vi "Test App Prefix Update is Propagated to Owned Processes.vi"(8 "error in (no error)":errorcluster, 11 "Application Test in":refnum<class "Application Dev Test.lvclass">) -> (0 "error out":errorcluster, 3 "Application Test out":refnum<class "Application Dev Test.lvclass">)   [LabVIEW 2020, in "Application Dev Test.lvclass"]
uses:
  Application Dev Test.lvclass
  C:/Program Files (x86)/National Instruments/LabVIEW 2020/vi.lib/Astemes/LUnit/Test Case.lvclass
  source/Framework/Application/Application.lvclass
  C:/Git/astemes-triarc-framework/source/Framework/Process/Process.lvclass
  source/Framework/Process/Process.lvclass
  source/Framework/Process/Process.lvclass/Process.ctl
  source/Framework/Application/Application.lvclass/Application.ctl
  <vilib>/Astemes/LUnit/Test Case.lvclass/Test Case.ctl
  <vilib>/Astemes/LUnit/LUnit Assertion Result.lvclass/LUnit Assertion Result.ctl
  <vilib>/Astemes/LUnit/LUnit Test Case Result.lvclass/LUnit Test Case Result.ctl
  <vilib>/Astemes/LUnit/LUnit Method Result.lvclass/LUnit Method Result.ctl
  source/Framework/Application/Private/Add Process to Map.vi
  source/Framework/Application/Private/Start Idle Processes if Running.vi
  source/Framework/Application/Private/Throw Error If Process Already in App.vi
  source/Framework/Process/Protected/Messaging/Enqueue Message.vi
  source/Framework/Process/Public/Lifecycle/Get Lifecycle State.vi
  source/Framework/Process/Protected/SubVIs/Set Context.vi
  source/Framework/Application/Private/Retrieve Process from App.vi
  source/Framework/Application/Private/Parse Process Name.vi
  source/Framework/Application/Private/Get Process from Map.vi
  <vilib>/Astemes/LUnit/Palette/Pass If Equal.vi/cbf50e99-f124-4847-863a-8e9794d3dede.vi
  source/Framework/Process/Private/SubVIs/Wait for finish.vi
  source/Framework/Process/Private/SubVIs/Set Lifecycle State.vi
  source/Framework/Process/Private/SubVIs/Handle Debug Data.vi
  <vilib>/Utility/error.llb/Clear Errors.vi
  source/Framework/Process/Public/Lifecycle/Leave Process Loop.vi
  source/Framework/Process/Protected/Messaging/Request Message.vi
  <vilib>/AdvancedString/Delimited String to 1D String Array.vi
  <vilib>/Astemes/LUnit/Palette/Pass.vi
  <vilib>/Astemes/LUnit/Palette/Fail.vi
  <vilib>/Astemes/LUnit/Compare Variants.vi
  <vilib>/Astemes/LUnit/Describe Comparison.vi
  <vilib>/Astemes/LUnit/Set Assertion Type.vi
  source/Framework/Logging/Log Debug.vi
  <vilib>/AdvancedString/1D String Array to Delimited String.vi
  <vilib>/Utility/High Resolution Relative Seconds.vi
  source/Framework/Process/Private/SubVIs/Enqueue Request Message.vi
  <vilib>/Astemes/LUnit/Add test result.vi
  <vilib>/Astemes/LUnit/LUnit Write Passed.vi
  <vilib>/Astemes/LUnit/LUnit Write Message.vi
  <vilib>/Astemes/LUnit/LUnit Write Description.vi
  <vilib>/Astemes/LUnit/Variant to string.vi
  <vilib>/Astemes/LUnit/LUnit Write Assertion Type.vi
  <vilib>/Astemes/LUnit/LUnit Record Assertion Result.vi
  <vilib>/Astemes/LUnit/LUnit Aggregate Assertion Results.vi
  <vilib>/Astemes/LUnit/Assertion Result/LUnit Read Status.vi
  <vilib>/Astemes/LUnit/LUnit Read Message.vi
  <vilib>/Astemes/LUnit/LUnit Read Description.vi
  <vilib>/Astemes/LUnit/Method Result/LUnit Merge Status.vi
  <vilib>/Astemes/LUnit/LUnit Concatenate result strings.vi
  <vilib>/Utility/error.llb/Error Cluster From Error Code.vi
  source/Framework/Process/Private/SubVIs/Wait for Response Message.vi
  <vilib>/Utility/Data Type/Get Type Information.vi
  <vilib>/Utility/LVClass/Get LV Class Name.vi
  <vilib>/Astemes/LUnit/LUnit Assertion Result.lvclass
  Application Dev Test.lvclass/Application Dev Test.ctl
  <vilib>/Astemes/LUnit/Test Case.lvclass
  source/Framework Test Suite/Support/Framework Test Support.lvlib
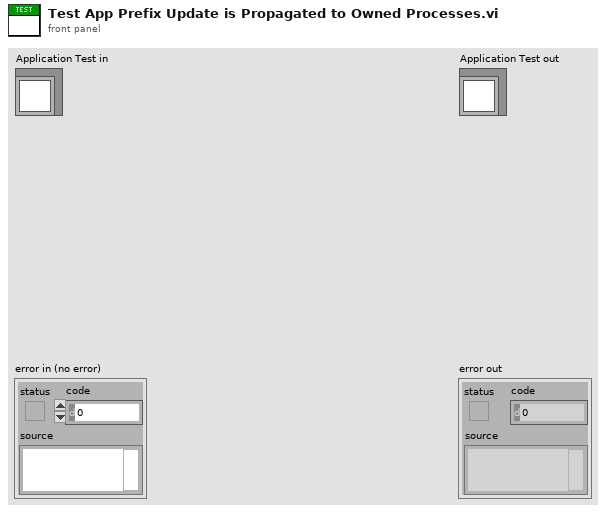
[diagram p1: front panel]
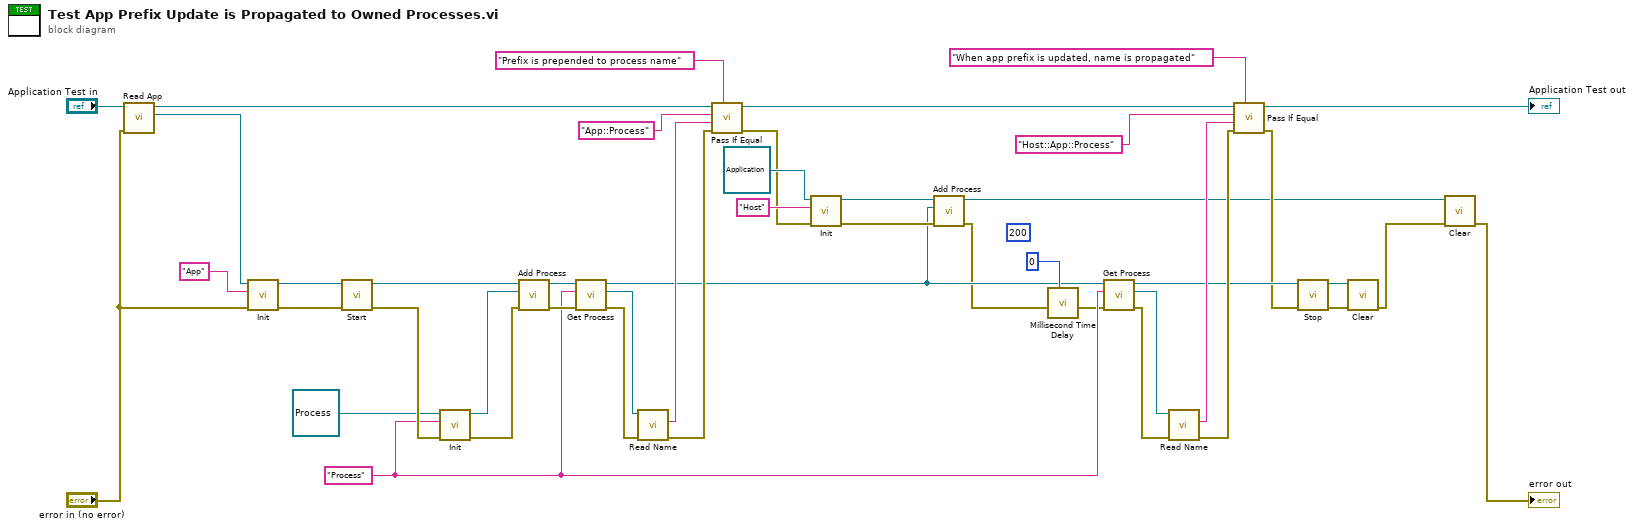
[diagram p0: block diagram]
diagram:
  (unwired) u32 200 ("milliseconds to wait")
  w21 = "Process" ("Name")
  n1 = call "Read App.vi"("error in (no error)"="error in (no error)", "Application Test In"="Application Test in") -> ("App out"=w12:refnum<class "Application.lvclass">, "Application Test Out"=w44:refnum<class "Application Dev Test.lvclass">)  [unwired: 7 in, 1 out]
  n2 = call-dynamic "Init.vi"("error in (no error)"="error in (no error)", "Name"="App", "Process In"=w12) -> ("error out"=w41:errorcluster, "Process Out"=w42:refnum<class "Application.lvclass">)  [unwired: 7 in]
  n3 = call "Start.vi"("error in (no error)"=w41, "Process In"=w42) -> ("error out"=w32:errorcluster, "Process Out"=w40:refnum<class "Application.lvclass">)  [unwired: 7 in, 1 out]
  n4 = call-dynamic "Init.vi"("error in (no error)"=w32, "Name"=w21, "Process In"=refnum<class "Process.lvclass"> refnum) -> ("error out"=w31:errorcluster, "Process Out"=w36:refnum<class "Process.lvclass">)  [unwired: 7 in]
  n5 = call "Add Process.vi"("error in (no error)"=w31, "Process"=w36, "Application In"=w40) -> ("error out"=w35:errorcluster, "Application Out"=w39:refnum<class "Application.lvclass">)  [unwired: 7 in]
  n6 = call "Get Process.vi"("error in (no error)"=w35, "Process Name"=w21, "Application In"=w39) -> ("error out"=w29:errorcluster, "App Process"=w30:refnum<class "Process.lvclass">, "Application Out"=w4:refnum<class "Application.lvclass">)  [unwired: 6 in]
  n7 = call "Read Name.vi"("error in (no error)"=w29, "Process In"=w30) -> ("error out"=w28:errorcluster, "Qualified Name"=w27:string)  [unwired: 6 in, 2 out]
  n8 = call <vilib>:"Pass If Equal.vi"("Description"="Prefix is prepended to process name", "error in (no error)"=w28, "Actual"=w27, "Expected"="App::Process", "LUnit Test Case In"=w44) -> ("error out"=w9:errorcluster, "LUnit Test Case Out"=w34:refnum<class "Application Dev Test.lvclass">)  [unwired: 5 in]
  n9 = call-dynamic "Init.vi"("error in (no error)"=w9, "Name"="Host" ("Prefix"), "Process In"=refnum<class "Application.lvclass"> refnum ("Rig In")) -> ("error out"=w7:errorcluster, "Process Out"=w8:refnum<class "Application.lvclass">)  [unwired: 7 in]
  n10 = call "Add Process.vi"("error in (no error)"=w7, "Process"=w4, "Application In"=w8) -> ("error out"=w3:errorcluster, "Application Out"=w6:refnum<class "Application.lvclass">)  [unwired: 7 in]
  n11 = call "Millisecond Time Delay.vi"("milliseconds to wait"=u32 0, "error in (no error)"=w3) -> ("error out"=w17:errorcluster)  [unwired: 7 in]
  n12 = call "Get Process.vi"("error in (no error)"=w17, "Process Name"=w21, "Application In"=w4) -> ("error out"=w23:errorcluster, "App Process"=w24:refnum<class "Process.lvclass">, "Application Out"=w14:refnum<class "Application.lvclass">)  [unwired: 6 in]
  n13 = call "Read Name.vi"("error in (no error)"=w23, "Process In"=w24) -> ("error out"=w18:errorcluster, "Qualified Name"=w22:string)  [unwired: 6 in, 2 out]
  n14 = call <vilib>:"Pass If Equal.vi"("Description"="When app prefix is updated, name is propagated", "error in (no error)"=w18, "Actual"=w22, "Expected"="Host::App::Process", "LUnit Test Case In"=w34) -> ("error out"=w13:errorcluster, "LUnit Test Case Out"=→"Application Test out":refnum<class "Application Dev Test.lvclass">)  [unwired: 5 in]
  n15 = call "Stop.vi"("error in (no error)"=w13, "Process In"=w14) -> ("error out"=w37:errorcluster, "Process Out"=w38:refnum<class "Application.lvclass">)  [unwired: 7 in, 1 out]
  n16 = call-dynamic "Clear.vi"("error in (no error)"=w37, "Application In"=w38) -> ("error out"=w2:errorcluster)  [unwired: 9 in]
  n17 = call-dynamic "Clear.vi"("error in (no error)"=w2, "Application In"=w6) -> ("error out"=→"error out":errorcluster)  [unwired: 9 in]
